vi "Create Gradient Color by Start Color and End Color.vi"(8 "错误输入":errorcluster, 9 "Length":i32=256, 10 "End":u32(colorbox), 11 "Start":u32(colorbox)) -> (0 "错误输出":errorcluster, 3 "ColorArray":u32[](array[colorbox]))   [LabVIEW 2012, in "Listbox Tool.lvlib"]
uses:
  <vilib>/Analysis/1siggen.llb/Ramp Pattern by Samples.vi
  Listbox Tool.lvlib
  <vilib>/Analysis/NI_AALBase.lvlib
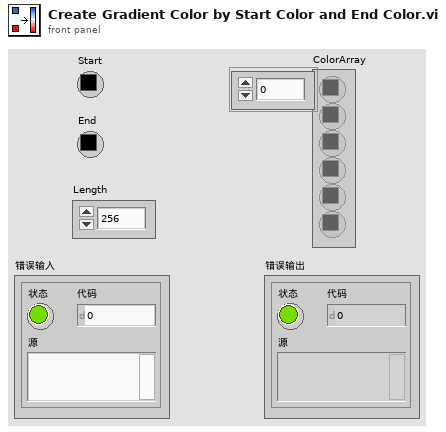
[diagram p1: front panel]
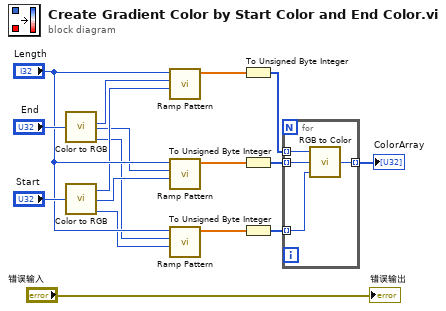
[diagram p0: block diagram]
diagram:
  n1 = call <vilib>:"Color to RGB.vi"("Color"="End") -> ("R"=w14:u8, "G"=w11:u8, "B"=w9:u8)  [unwired: 1 out]
  n2 = call <vilib>:"Color to RGB.vi"("Color"="Start") -> ("R"=w12:u8, "G"=w10:u8, "B"=w8:u8)  [unwired: 1 out]
  n3 = call-poly <vilib>:"Ramp Pattern.vi"("start"=w12, "end"=w14, "samples"="Length") -> ("Ramp Pattern"=w7:dbl[])  [unwired: 7 in, 1 out]
  n4 = call-poly <vilib>:"Ramp Pattern.vi"("start"=w10, "end"=w11, "samples"="Length") -> ("Ramp Pattern"=w6:dbl[])  [unwired: 7 in, 1 out]
  n5 = call-poly <vilib>:"Ramp Pattern.vi"("start"=w8, "end"=w9, "samples"="Length") -> ("Ramp Pattern"=w5:dbl[])  [unwired: 7 in, 1 out]
  n6 = To Unsigned Byte Integer(number=w7) -> (unsigned 8bit integer=w4:u8[])
  n7 = To Unsigned Byte Integer(number=w6) -> (unsigned 8bit integer=w3:u8[])
  n8 = To Unsigned Byte Integer(number=w5) -> (unsigned 8bit integer=w2:u8[])
  n9 = for {
    tunnel: w4 -> [w21] mode=indexing
    tunnel: w3 -> [w20] mode=indexing
    tunnel: w2 -> [w19] mode=indexing
    tunnel: [w18] -> w1 mode=indexing
    n10 = call <vilib>:"RGB to Color.vi"("B"=w19, "G"=w20, "R"=w21) -> ("Color"=w18:u32)
  }
  "ColorArray" <- w1
  "错误输出" <- "错误输入"
